vi "test.vi"() -> ()   [LabVIEW 2024]
panel:
  in  "OK Button":bool
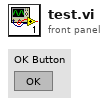
[diagram p1: front panel]
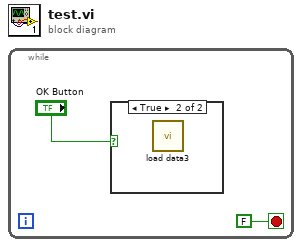
[diagram p0: block diagram]
diagram:
  n1 = while {
    stop <- FALSE stop-if-true
    n2 = case shown="True" "OK Button" {
      frame False {
      }
      frame True {
        n3 = call "load data3.vi"() -> ()  [unwired: 10 in, 2 out]
      }
    }
  }
